vi "Write.vi"(6 "Append Index":i32, 8 "error in (no error)":errorcluster, 9 "Notes":string, 10 "Data (Dictionary)":T1[](array[typedef]), 11 "Data in":refnum<class "Data.lvclass">) -> (0 "error out":errorcluster, 3 "Data out":refnum<class "Data.lvclass">, 5 "Path out":path)   [LabVIEW 2016, in "Data.lvclass"]
uses:
  Data.lvclass
  Typedefs/Dictionary--cluster.ctl
  Data.lvclass/Data.ctl
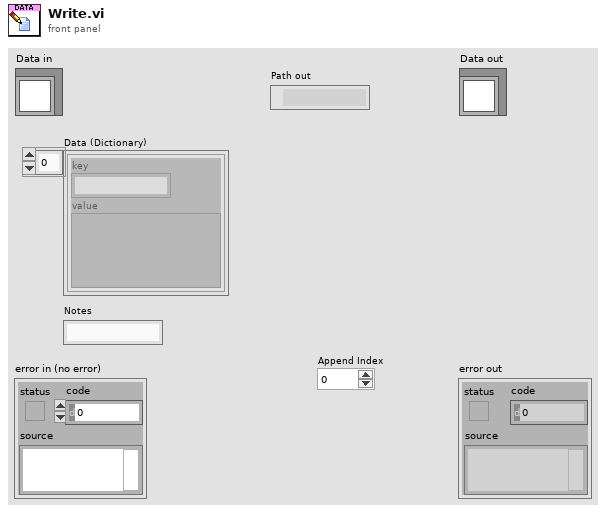
[diagram p1: front panel]
types:
  T1 = typedef "Data.lvclass/Dictionary--cluster.ctl" = cluster{"key":string, "value":variant}
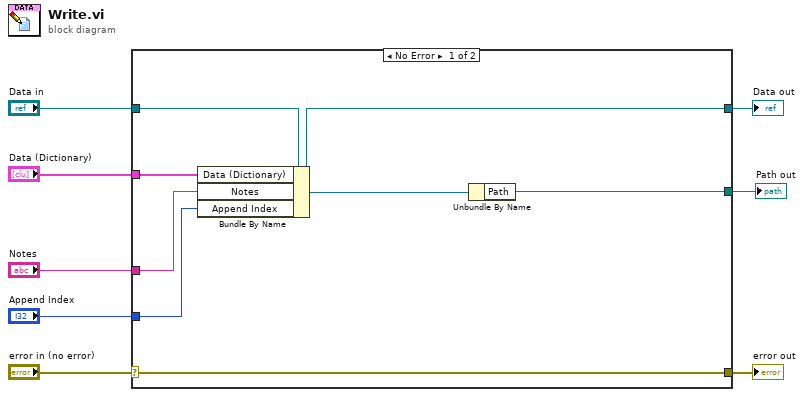
[diagram p0: block diagram]
diagram:
  n1 = case shown="No Error" "error in (no error)" {
    selector: "error in (no error)" -> [w10 w17]
    tunnel: [w10 w17] -> w7
    tunnel: [w9 w16] -> w5
    tunnel: "Data in" -> [w12 w16]
    tunnel: [w15 _] -> w4
    tunnel: "Data (Dictionary)" -> [w14 _]
    tunnel: "Notes" -> [w13 _]
    tunnel: "Append Index" -> [w11 _]
    frame No Error {
      n2 = Bundle By Name(cluster=w12, "Data (Dictionary)"=w14, "Notes"=w13, "Append Index"=w11) -> (w9:refnum<class "Data.lvclass">)
      n3 = Unbundle By Name(w9) -> ("Path"=w15:path)
    }
    frame Error {
    }
  }
  "error out" <- w7
  "Data out" <- w5
  "Path out" <- w4
